vi "Clusterwitharrayerrcluster.vi"(1 "Cluster In":T2) -> (0 "Cluster Out":T1)   [LabVIEW 2010]
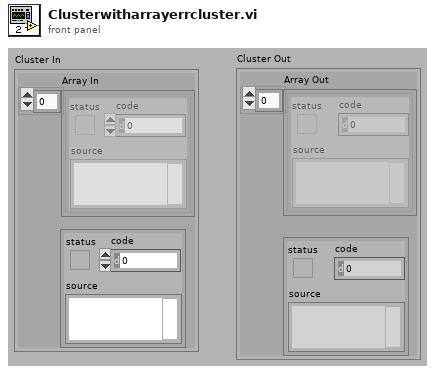
[diagram p1: front panel]
types:
  T1 = cluster{"Array Out":errorcluster[], "error out":errorcluster}
  T2 = cluster{"Array In":errorcluster[], "error in (no error)":errorcluster}
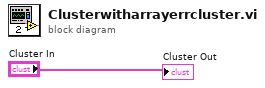
[diagram p0: block diagram]
diagram:
  "Cluster Out" <- "Cluster In"
